vi "FGV.vi"(9 "Comandos":string, 10 "Respuestas":string, 11 "Función":T1(ring)) -> (1 "Respuesta":string)   [LabVIEW 2020, in "Simulado.lvclass"]
uses:
  Simulado.lvclass
panel:
  out "Variant":variant
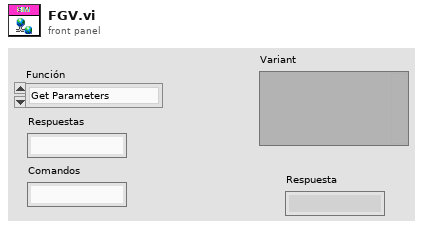
[diagram p1: front panel]
types:
  T1 = enum16{"Get Parameters", "Set Parameters", "Reset"}
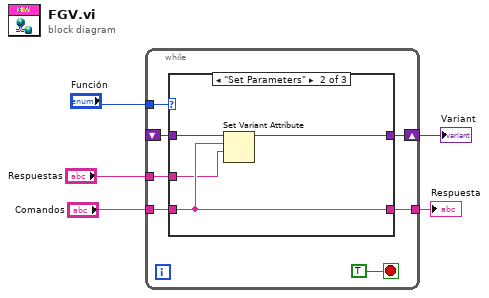
[diagram p0: block diagram]
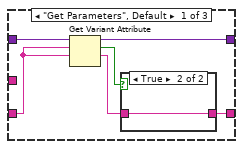
[diagram p2: hidden frame]
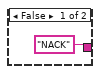
[diagram p3: hidden frame]
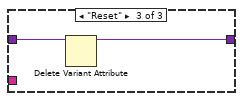
[diagram p4: hidden frame]
diagram:
  n1 = while {
    tunnel: "Función" -> [w11]
    shift-right: [w10] -> w4
    shift-left: _ -> [w9]
    tunnel: "Respuestas" -> [w8]
    tunnel: [w7] -> w3
    tunnel: "Comandos" -> [w6]
    stop <- TRUE stop-if-true
    n2 = case shown="\"Set Parameters\"" w11 {
      tunnel: [w18 w23 w25] -> w10
      tunnel: w9 -> [w17 w24 w26]
      tunnel: w8 -> [_ w21 _]
      tunnel: [w15 w22 _] -> w7
      tunnel: w6 -> [w13 w22 _]
      frame "Get Parameters", Default {
        n3 = Get Variant Attribute(Variant=w17, name=w13, default value (empty Variant)=w13) -> (duplicate Variant=w18:variant, found=w16:bool, value=w14:string)  [unwired: 1 in, 1 out]
        n4 = case shown="True" w16 {
          tunnel: ["NACK" w20] -> w15
          tunnel: w14 -> [_ w20]
          frame False {
          }
          frame True {
          }
        }
      }
      frame "Set Parameters" {
        n5 = Set Variant Attribute(Variant=w24, name=w22, value=w21) -> (Variant out=w23:variant)  [unwired: 1 in, 2 out]
      }
      frame "Reset" {
        n6 = Delete Variant Attribute(7:w26) -> (3:w25:variant)  [unwired: 2 in, 2 out]
      }
    }
  }
  "Respuesta" <- w3
  "Variant" <- w4
